vi "DigitalWrite.vi"(8 "error in (no error)":errorcluster, 10 "on/off":bool, 11 "lines":tag="Dev3/port0/line0") -> (0 "error out":errorcluster)   [LabVIEW 2018]
uses:
  <vilib>/DAQmx/write.llb/DAQmx Write (Digital Bool 1Line 1Point).vi
  <vilib>/DAQmx/create/channels.llb/DAQmx Create Channel (DO-Digital Output).vi
  <vilib>/DAQmx/miscellaneous.llb/DAQmx Fill In Error Info.vi
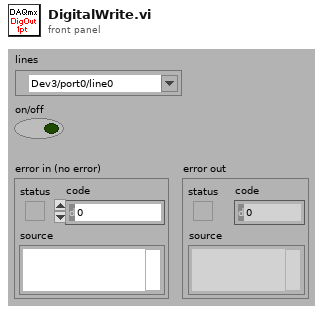
[diagram p1: front panel]
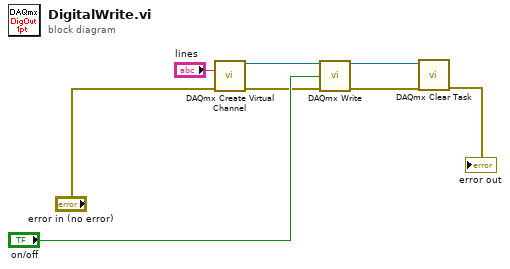
[diagram p0: block diagram]
diagram:
  n1 = call-poly <vilib>:"DAQmx Create Virtual Channel.vi"("lines"="lines", "error in"="error in (no error)") -> ("task out"=w7:refnum<k21>, "error out"=w3:errorcluster)  [unwired: 12 in]
  n2 = call-poly <vilib>:"DAQmx Write.vi"("task/channels in"=w7, "data"="on/off", "error in"=w3) -> ("task out"=w5:refnum<k21>, "error out"=w2:errorcluster)  [unwired: 10 in, 1 out]
  n3 = call <vilib>:"DAQmx Clear Task.vi"("task in"=w5, "error in"=w2) -> ("error out"=→"error out":errorcluster)  [unwired: 13 in]
